vi "test Read Multiple Event Registration.vi"(11 "Test Case In":refnum<class "Tests Event MessengerM.lvclass">) -> (0 "error out":errorcluster, 3 "Test Case Out":refnum<class "Tests Event MessengerM.lvclass">)   [LabVIEW 2020, in "Tests Event MessengerM.lvclass"]
uses:
  Tests Event MessengerM.lvclass
  C:/Program Files/National Instruments/LabVIEW 2025/vi.lib/Astemes/LUnit/Test Case.lvclass
  <vilib>/Astemes/LUnit/Test Case.lvclass/Test Case.ctl
  <vilib>/Astemes/LUnit/Test Case.lvclass
  <extravilib>/ChannelInstances/Event MessengerM-c(str,var).lvlib
panel:
  out "Array 2":string[](array[string])
  out "Array":string[](array[string])
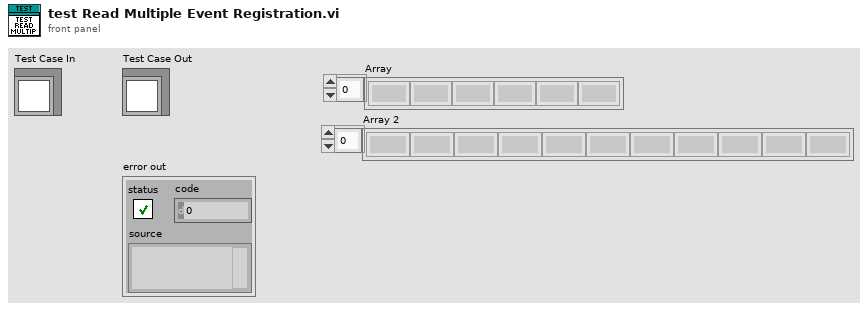
[diagram p1: front panel]
types:
  T1 = typedef "Event MessengerM-c(str,var).lvlib/))Channel.ctl" = refnum<queue>
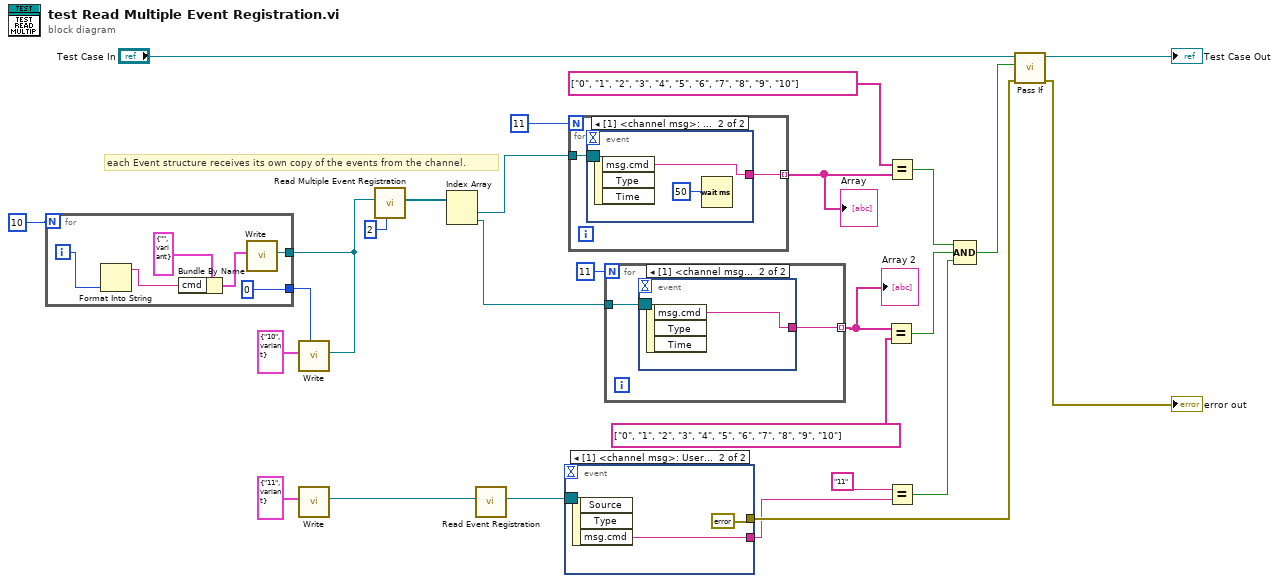
[diagram p0: block diagram]
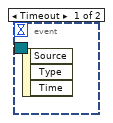
[diagram p2: hidden frame]
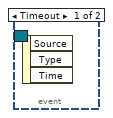
[diagram p3: hidden frame]
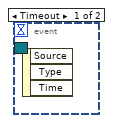
[diagram p4: hidden frame]
diagram:
  # "each Event structure receives its own copy of the events from the channel."
  n1 = for {
    N: 10 -> [_]
    tunnel: [w29] -> w14
    tunnel: [0] -> w6
    i -> [w32]
    n2 = Format Into String(w32) -> (resulting string=w31:string)  [unwired: 3 in, 1 out]
    n3 = Bundle By Name(cluster=cluster{"cmd":string, "data":variant} {"cmd"="", "data"=variant} ("element"), "cmd"=w31) -> (w30:cluster{"cmd":string, "data":variant})
    n4 = call <extravilib>:"Write.vi"("element"=w30) -> ("channel"=w29:T1)  [unwired: 9 in, 1 out]
  }
  n5 = call <extravilib>:"Write.vi"("channel"=w14, "subchannel (0)"=w6, "element"=cluster{"cmd":string, "data":variant} {"cmd"="10", "data"=variant}) -> ()  [unwired: 8 in, 1 out]
  n6 = call <extravilib>:"Write.vi"("element"=cluster{"cmd":string, "data":variant} {"cmd"="11", "data"=variant}) -> ("channel"=w10:T1)  [unwired: 9 in, 1 out]
  n7 = call <extravilib>:"Read Multiple Event Registration.vi"("number of event structures"=u16 2, "channel in"=w14) -> ("event registration refnums"=w13:refnum<event-registration>[])  [unwired: 9 in]
  n8 = Index Array(array=w13) -> (element #1=w17:refnum<event-registration>, element #2=w16:refnum<event-registration>)  [unwired: 2 in]
  n9 = call <extravilib>:"Read Event Registration.vi"("channel"=w10) -> ("event registration refnum"=w9:refnum<event-registration>)  [unwired: 10 in]
  n10 = event shown="[1] <channel msg>: User Event" {
    selector: w9 -> [_ _]
    dyn-events: _ -> [_ _]
    timeout: _ -> [_ _]
    tunnel: [_ errorcluster {"status"=FALSE, "code"=0, "source"=""} ("error constant")] -> w18
    tunnel: [_ w34] -> w5
    event Timeout {
      n11 = event-data() -> ()  [unwired: 1 in, 3 out]
    }
    event User Event {
      n12 = event-data() -> ("msg.cmd"=w34:string)  [unwired: 1 in, 2 out]
    }
  }
  n13 = for {
    N: 11 -> [_]
    tunnel: w17 -> [w36]
    tunnel: [w37] -> w8 mode=indexing
    n14 = event shown="[1] <channel msg>: User Event" {
      selector: w36 -> [_ _]
      dyn-events: _ -> [_ _]
      timeout: _ -> [_ _]
      tunnel: [_ w39] -> w37
      event Timeout {
        n15 = event-data() -> ()  [unwired: 1 in, 3 out]
      }
      event User Event {
        n16 = event-data() -> ("msg.cmd"=w39:string)  [unwired: 1 in, 2 out]
        n17 = Wait (ms)(milliseconds to wait=u32 50) -> ()  [unwired: 1 out]
      }
    }
  }
  "Array" <- w8
  n18 = for {
    N: 11 -> [_]
    tunnel: [w41] -> w7 mode=indexing
    tunnel: w16 -> [w40]
    n19 = event shown="[1] <channel msg>: User Event" {
      selector: w40 -> [_ _]
      dyn-events: _ -> [_ _]
      timeout: _ -> [_ _]
      tunnel: [_ w42] -> w41
      event Timeout {
        n20 = event-data() -> ()  [unwired: 1 in, 3 out]
      }
      event User Event {
        n21 = event-data() -> ("msg.cmd"=w42:string)  [unwired: 1 in, 2 out]
      }
    }
  }
  "Array 2" <- w7
  n22 = Equal?(x=w7, y=string[] ["0", "1", "2", "3", "4", "5", "6", "7", "8", "9", "10"] ("Array 2")) -> (x = y?=w21:bool)
  n23 = Equal?(x=string[] ["0", "1", "2", "3", "4", "5", "6", "7", "8", "9", "10"] ("Array 2"), y=w8) -> (x = y?=w20:bool)
  n24 = Equal?(x="11", y=w5) -> (x = y?=w3:bool)
  n25 = Compound Arithmetic op=AND(w20, w21, w3) -> (w19:bool)
  n26 = call <vilib>:"Pass If.vi"("error in (no error)"=w18, "Pass?"=w19, "LUnit Test Case In"="Test Case In") -> ("error out"=→"error out":errorcluster, "LUnit Test Case Out"=→"Test Case Out":refnum<class "Tests Event MessengerM.lvclass">)  [unwired: 7 in]
